vi "Read Script Name.vi"(11 "Build Job in":refnum<class "Build Job.lvclass">) -> (2 "Script Name":string)   [LabVIEW 2014, in "Build Job.lvclass"]
uses:
  Build Job.lvclass
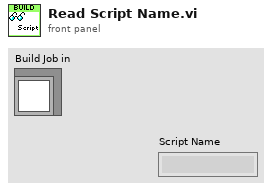
[diagram p1: front panel]
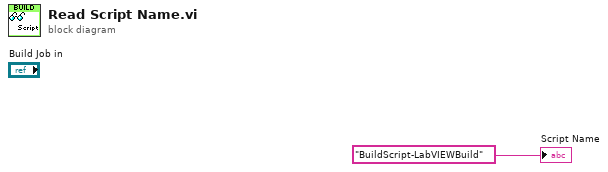
[diagram p0: block diagram]
diagram:
  "Script Name" <- "BuildScript-LabVIEWBuild" ("Script Job Name")
